vi "Angle.vi"(7 "Vertex":cluster{"Xv":dbl, "Yv":dbl}, 10 "Object":cluster{"X":sgl, "Y":sgl}, 11 "initial":cluster{"X0":sgl, "Y0":sgl}) -> (2 "Angle raw":dbl, 3 "Angle modified":dbl)   [LabVIEW 2019]
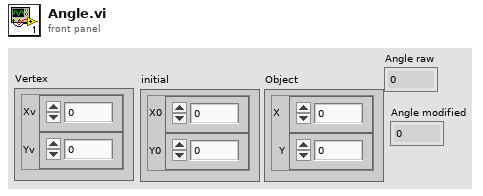
[diagram p1: front panel]
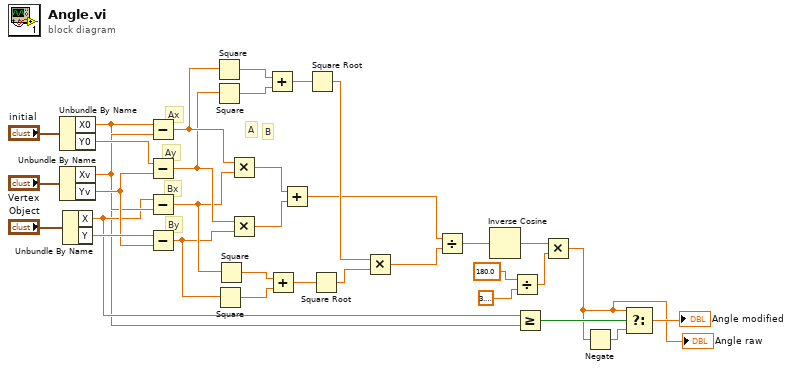
[diagram p0: block diagram]
diagram:
  # "By"
  # "Bx"
  # "Ay"
  # "Ax"
  # "B"
  # "A"
  n1 = Unbundle By Name("initial") -> ("X0"=w5:sgl, "Y0"=w30:sgl)
  n2 = Unbundle By Name("Vertex") -> ("Xv"=w28:dbl, "Yv"=w29:dbl)
  n3 = Unbundle By Name("Object") -> ("X"=w6:sgl, "Y"=w31:sgl)
  n4 = Subtract(x=w5, y=w28) -> (x-y=w11:dbl)
  n5 = Subtract(x=w30, y=w29) -> (x-y=w10:dbl)
  n6 = Subtract(x=w6, y=w28) -> (x-y=w9:dbl)
  n7 = Subtract(x=w31, y=w29) -> (x-y=w8:dbl)
  n8 = Square(x=w11) -> (x^2=w25:dbl)
  n9 = Square(x=w10) -> (x^2=w24:dbl)
  n10 = Square(x=w8) -> (x^2=w22:dbl)
  n11 = Square(x=w9) -> (x^2=w23:dbl)
  n12 = Multiply(x=w11, y=w9) -> (x*y=w27:dbl)
  n13 = Multiply(x=w10, y=w8) -> (x*y=w26:dbl)
  n14 = Add(x=w25, y=w24) -> (x+y=w20:dbl)
  n15 = Add(x=w23, y=w22) -> (x+y=w21:dbl)
  n16 = Add(x=w27, y=w26) -> (x+y=w7:dbl)
  n17 = Square Root(x=w20) -> (sqrt(x)=w19:dbl)
  n18 = Square Root(x=w21) -> (sqrt(x)=w18:dbl)
  n19 = Multiply(x=w19, y=w18) -> (x*y=w17:dbl)
  n20 = Divide(x=w7, y=w17) -> (x/y=w16:dbl)
  n21 = Inverse Cosine(1:w16) -> (0:w13:dbl)
  n22 = Divide(x=180.0, y=3.141592653589793) -> (x/y=w12:dbl)
  n23 = Greater Or Equal?(x=w6, y=w5) -> (x >= y?=w4:bool)
  n24 = Multiply(x=w13, y=w12) -> (x*y=w1:dbl)
  "Angle raw" <- w1
  n25 = Negate(x=w1) -> (-x=w3:dbl)
  n26 = Select(t=w1, s=w4, f=w3) -> (s? t:f=→"Angle modified":dbl)
